vi "SL TAGS Return Interpolation Method.vi"(4 "Interpolation Method":T1) -> (1 "Seeq Interpolation Method":string)   [LabVIEW 2017, in "EEISysLink.lvclass"]
doc: "Convert selected interpolation method to Seeq supported interpolation method string\n\nJames Tillett\nEndeavor Engineering Inc.\nwww.endeavoreng.com"
uses:
  EEISysLink.lvclass
  Controls/SL Tag Interpolation Method.ctl
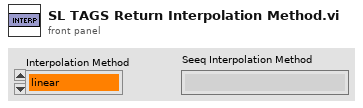
[diagram p1: front panel]
types:
  T1 = typedef "EEISysLink.lvclass/SL Tag Interpolation Method.ctl" = enum16{"linear", "pilinear", "step"}
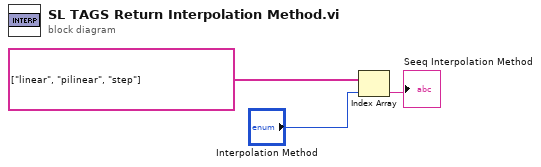
[diagram p0: block diagram]
diagram:
  n1 = Index Array(array=string[] ["linear", "pilinear", "step"], index="Interpolation Method") -> (element=→"Seeq Interpolation Method":string)
